vi "TDT-Set Multiplexer.vi"(0 "RPcox":refnum<k7>, 5 "iAzimuth":i32, 7 "MUX 1":i32, 9 "MUX 2":i32, 11 "error in (no error)":errorcluster) -> (4 "RPcox thru":refnum<k7>, 15 "error out":errorcluster)   [LabVIEW 2020]
panel:
  out "WordOut":u8[](array[numeric]) format="%08b"
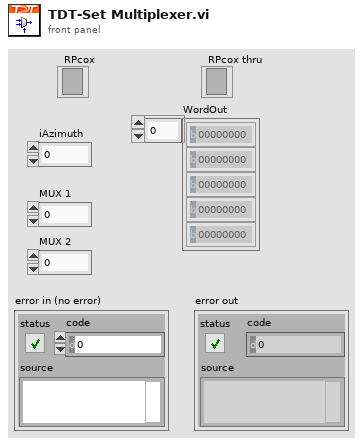
[diagram p1: front panel]
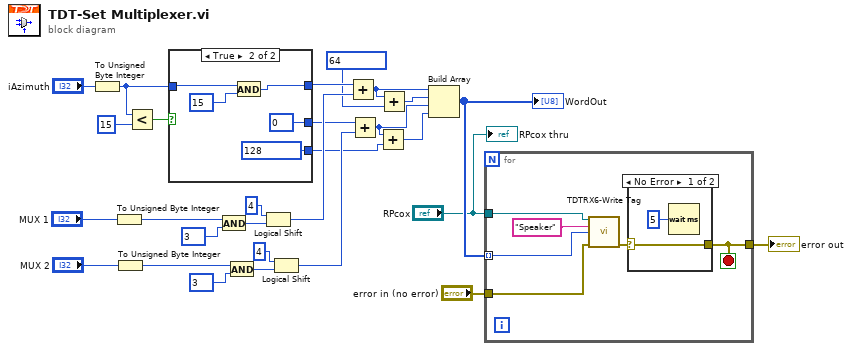
[diagram p0: block diagram]
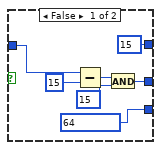
[diagram p3: hidden frame]
diagram:
  n1 = To Unsigned Byte Integer(number="iAzimuth") -> (unsigned 8bit integer=w25:u8)
  n2 = To Unsigned Byte Integer(number="MUX 1") -> (unsigned 8bit integer=w19:u8)
  n3 = To Unsigned Byte Integer(number="MUX 2") -> (unsigned 8bit integer=w15:u8)
  n4 = Less?(x=w25, y=u8 15) -> (x < y?=w27:bool)
  n5 = case shown="True" w27 {
    tunnel: w25 -> [w34 w40]
    tunnel: [u8 15 ("y") w38] -> w14
    tunnel: [w30 u8 0 ("y")] -> w12
    tunnel: [u8 64 ("y") u8 128 ("y")] -> w3
    frame False {
      n6 = Subtract(x=w34, y=u8 15) -> (x-y=w31:u8)
      n7 = And(x=w31, y=u8 15) -> (x .and. y?=w30:u8)
    }
    frame True {
      n8 = And(x=w40, y=u8 15) -> (x .and. y?=w38:u8)
    }
  }
  n9 = And(x=w19, y=u8 3) -> (x .and. y?=w21:u8)
  n10 = And(x=w15, y=u8 3) -> (x .and. y?=w17:u8)
  n11 = Logical Shift(y=i16 4, x=w21) -> (x << y=w13:u8)
  n12 = Logical Shift(y=i16 4, x=w17) -> (x << y=w11:u8)
  n13 = Add(x=w14, y=w13) -> (x+y=w5:u8)
  n14 = Add(x=w12, y=w11) -> (x+y=w4:u8)
  n15 = Add(x=w4, y=w3) -> (x+y=w2:u8)
  n16 = Add(x=w5, y=u8 64) -> (x+y=w7:u8)
  n17 = Build Array(w5, w7, w4, w2) -> (w10:u8[])
  "WordOut" <- w10
  n18 = for {
    tunnel: w10 -> [w45] mode=indexing
    tunnel: "error in (no error)" -> [w44]
    tunnel: [w42] -> w8
    tunnel: "RPcox" -> [w41]
    stop <- w42 stop-if-true
    n19 = call "TDTRX6-Write Tag.vi"("RPcox"=w41, "Name"="Speaker", "Value"=w45, "error in"=w44) -> ("error out"=w43:errorcluster)  [unwired: 10 in, 1 out]
    n20 = case shown="No Error" w43 {
      selector: w43 -> [w48 w49]
      tunnel: [w48 w49] -> w42
      frame No Error {
        n21 = Wait (ms)(milliseconds to wait=u32 5) -> ()  [unwired: 1 out]
      }
      frame Error {
      }
    }
  }
  "error out" <- w8
  "RPcox thru" <- "RPcox"
